vi "Save Test Data.vi"(8 "error in (no error)":errorcluster, 10 "Test Data Array":waveform(dbl)[](array[waveform]), 11 "Platform in":refnum<class "Platform.lvclass">) -> (0 "error out":errorcluster, 3 "Platform out":refnum<class "Platform.lvclass">)   [LabVIEW 2019]
uses:
  Platform.lvclass
  C:/Program Files (x86)/National Instruments/LabVIEW 2019/vi.lib/MGI/Panel Manager/Panel Actor/Panel Actor/Panel Actor.lvclass
  C:/Program Files (x86)/National Instruments/LabVIEW 2019/vi.lib/MGI/Monitored Actor/Monitored Actor/Monitored Actor/Monitored Actor.lvclass
  C:/Program Files (x86)/National Instruments/LabVIEW 2019/vi.lib/ActorFramework/Actor/Actor.lvclass
  Platform Messages/Run Msg/PF Commands Msg.lvclass
  C:/Program Files (x86)/National Instruments/LabVIEW 2019/vi.lib/ActorFramework/Message/Message.lvclass
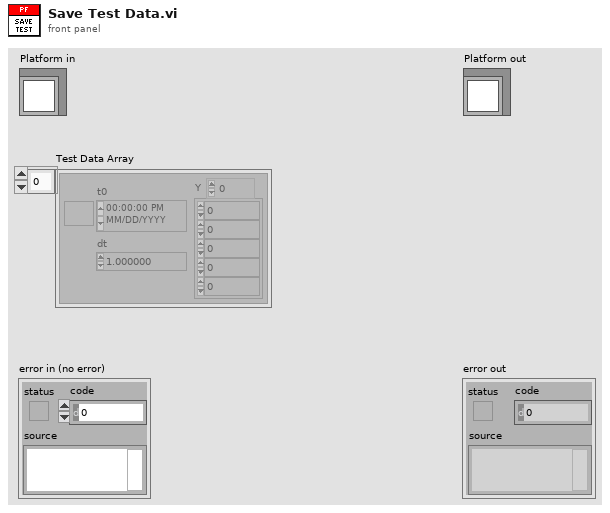
[diagram p1: front panel]
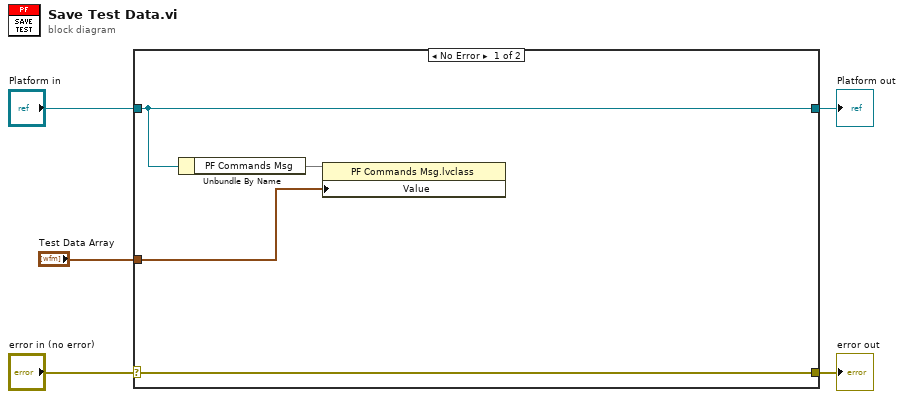
[diagram p0: block diagram]
diagram:
  n1 = case shown="No Error" "error in (no error)" {
    selector: "error in (no error)" -> [w9 w11]
    tunnel: [w9 w11] -> w4
    tunnel: [w7 w10] -> w2
    tunnel: "Platform in" -> [w7 w10]
    tunnel: "Test Data Array" -> [w6 _]
    frame No Error {
      n2 = Unbundle By Name(w7) -> ("PF Commands Msg"=w8)
      n3 = property class="PF Commands Msg.lvclass"(reference=w8, "Value"=w6) -> ()  [unwired: 1 in, 2 out]
    }
    frame Error {
    }
  }
  "error out" <- w4
  "Platform out" <- w2
